vi "Set Item Property.vi"(8 "error in (no error)":errorcluster, 9 "Value":variant, 10 "Property Name":string, 11 "Item Reference in":T1 format="%.0x") -> (0 "error out":errorcluster, 3 "Item Reference out":T1 format="%.0x", 4 "replaced":bool)   [LabVIEW 2013, in "Hierarchy Framework.lvlib" / "Item.lvclass"]
doc: "Sets a <B>Property Name</B> and <B>Value</B> for an item property and saves this information in the system definition file. If the <B>Property Name</B> you specify already exists, this VI overwrites the property. Wire data to the <B>Value</B> input to determine the polymorphic instance to use or manually select the instance."
uses:
  Item.lvclass
  Ctls/Item Reference.ctl
  Generic/Generic.lvclass
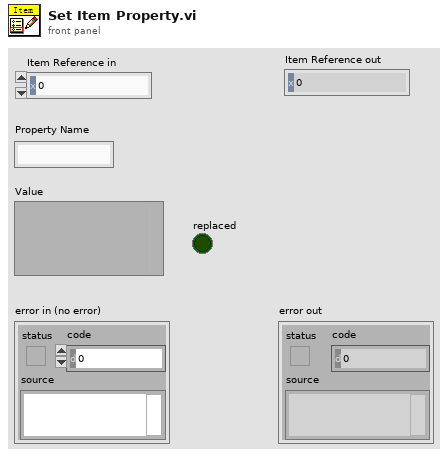
[diagram p1: front panel]
types:
  T1 = typedef "Hierarchy Framework.lvlib/Item.lvclass/Item Reference.ctl" = u64
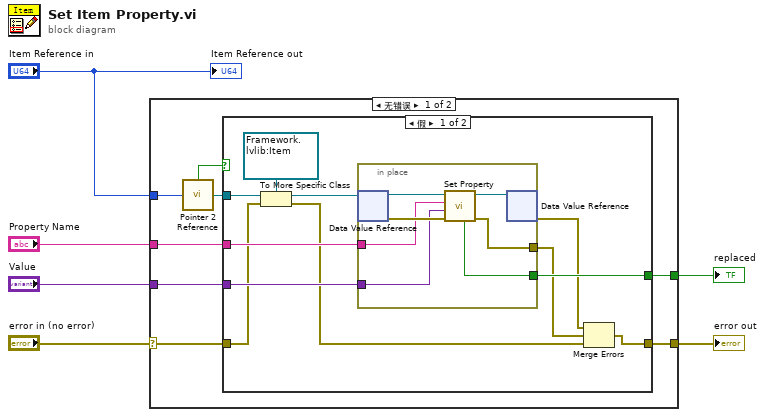
[diagram p0: block diagram]
diagram:
  n1 = case shown="无错误" "error in (no error)" {
    selector: "error in (no error)" -> [w8 w34]
    tunnel: "Item Reference in" -> [w11 _]
    tunnel: "Property Name" -> [w14 _]
    tunnel: "Value" -> [w13 _]
    tunnel: [w12 _] -> w3
    tunnel: [w7 w34] -> w1
    frame No Error {
      n2 = call "Pointer 2 Reference.vi"("Pointer"=w11) -> ("Not A Refnum?"=w10:bool, "Generic Reference"=w9:refnum<data-value>)
      n3 = case shown="假" w10 {
        tunnel: w9 -> [w22 _]
        tunnel: w14 -> [w25 _]
        tunnel: w13 -> [w24 _]
        tunnel: [w23 _] -> w12
        tunnel: w8 -> [w19 w33]
        tunnel: [w15 w33] -> w7
        frame False {
          n4 = To More Specific Class(target class=refnum<data-value> refnum ("Item"), reference=w22, error in=w19) -> (specific class reference=w20:refnum<data-value>, error out=w18:errorcluster)
          n5 = in-place {
            in-place-border: w25 -> [w30]
            in-place-border: w24 -> [w29]
            in-place-border: [w28] -> w23
            in-place-border: [w27] -> w16
            n6 = in-place-dvr #1(w20) -> (w26:refnum<class "Item.lvclass">, w31:errorcluster)
            n7 = call-dynamic "Set Property.vi"("error in (no error)"=w31, "Value"=w29, "Property Name"=w30, "Item输入"=w26) -> ("error out"=w27:errorcluster, "Item输出"=w32:refnum<class "Item.lvclass">, "replaced"=w28:bool)  [unwired: 5 in]
            n8 = in-place-dvr #1(w32) -> (w17:errorcluster)  [unwired: 1 out]
          }
          n9 = Merge Errors(w17, w16, w18) -> (w15:errorcluster)
        }
        frame True {
        }
      }
    }
    frame Error {
    }
  }
  "replaced" <- w3
  "error out" <- w1
  "Item Reference out" <- "Item Reference in"
